vi "Overwrite-all-hidden-parameters.vi"(8 "error in (no error)":errorcluster, 10 "Acquis params adv":T1={"Image acquisition timeout factor"=1.0, "Image collection timeout factor"=2.0, "Manual trigger ID"=25, "Precision hardware counter"="Dev1/ctr0", "When to use gate signal?"=FALSE, "Minimum acquisition timeout"=0, "External timing channel"="/Dev1/PFI4", "External gating channel"=""}, 11 "Acquis. params. ref. in":refnum<data-value>) -> (0 "error out":errorcluster, 3 "Acquis. params. ref.":refnum<data-value>)   [LabVIEW 2013, in "CameraVision.lvlib" / "CV-Acquisition.lvclass"]
uses:
  CV-Acquisition.lvclass
  Acquisition-parameters-advanced.ctl
  CV-Acquisition.lvclass/CV-Acquisition.ctl
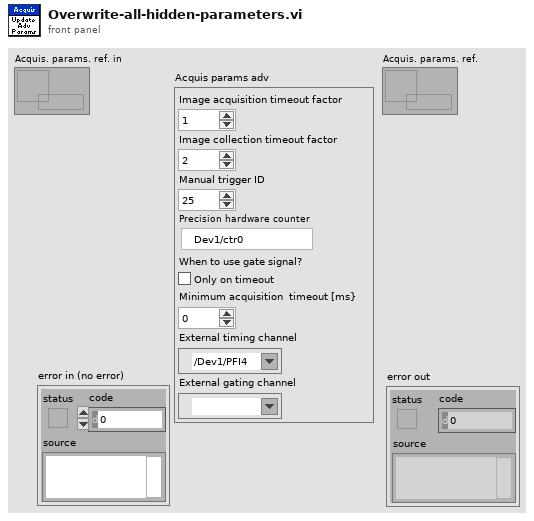
[diagram p1: front panel]
types:
  T1 = typedef "CameraVision.lvlib/CV-Acquisition.lvclass/Acquisition-parameters-advanced.ctl" = cluster{"Image acquisition timeout factor":dbl, "Image collection timeout factor":dbl, "Manual trigger ID":u8, "Precision hardware counter":tag, "When to use gate signal?":bool, "Minimum acquisition timeout":i32, "External timing channel":tag, "External gating channel":tag}
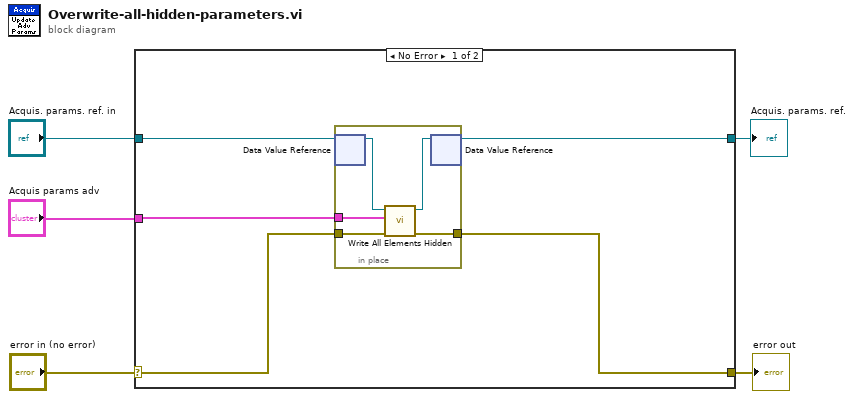
[diagram p0: block diagram]
diagram:
  n1 = case shown="No Error" "error in (no error)" {
    selector: "error in (no error)" -> [w6 w17]
    tunnel: [w10 w17] -> w4
    tunnel: "Acquis. params. ref. in" -> [w8 w16]
    tunnel: "Acquis params adv" -> [w9 _]
    tunnel: [w7 w16] -> w1
    frame No Error {
      n2 = in-place {
        in-place-border: [w15] -> w10
        in-place-border: w9 -> [w14]
        in-place-border: w6 -> [w12]
        n3 = in-place-dvr #1(w8) -> (w13:refnum<class "CV-Acquisition.lvclass">)  [unwired: 1 out]
        n4 = call "Write All Elements Hidden.vi"("error in (no error)"=w12, "Acquis. params. hidden"=w14, "Acquis params in"=w13) -> ("error out"=w15:errorcluster, "Acquis params out"=w11:refnum<class "CV-Acquisition.lvclass">)  [unwired: 7 in]
        n5 = in-place-dvr #1(w11) -> (w7:refnum<data-value>)  [unwired: 1 out]
      }
    }
    frame Error {
    }
  }
  "error out" <- w4
  "Acquis. params. ref." <- w1
